vi "breakout.vi"(11 "NXT/EV3":T1) -> (3 "NXT/EV3 2":T1)   [LabVIEW 2013]
uses:
  <vilib>/NXT/Subs/LVHSConnector.ctl
  <vilib>/NXT/LegoClasses/BrickReference/BrickReference.lvclass
  <vilib>/NXT/Dual Mode Library/Display/NXT_Rect.ctl
  <vilib>/NXT/Dual Mode Library/Display/clearDisplay.vi
  <vilib>/NXT/Dual Mode Library/Waits/Wait_Num.vi
  <vilib>/NXT/Dual Mode Library/prims/inRangeAndCoerce/inRangeAndCoerce_float.vi
  <vilib>/NXT/Dual Mode Library/Display/eraseRect.vi
  <vilib>/NXT/Dual Mode Library/Display/drawRect_filled.vi
  <vilib>/NXT/Dual Mode Library/Advanced/NXTFlag_Get_Integer.vi
  <vilib>/NXT/Dual Mode Library/Sensors/EV3_Infrared_Seek.vi
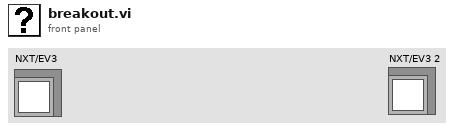
[diagram p1: front panel]
types:
  T1 = typedef "LVHSConnector.ctl" = refnum<class "BrickReference.lvclass">
  T2 = typedef "NXT_Rect.ctl" = cluster{"Left":i16, "Bottom":i16, "Width":i16, "Height":i16}
  T3 = cluster{dbl, dbl, "lower limit":i32, "lower limit":i32}
  T4 = cluster{"Channel 1 Heading":sgl, "Channel 1 Proximity":sgl, "Channel 2 Heading":sgl, "Channel 2 Proximity":sgl, "Channel 3 Heading":sgl, "Channel 3 Proximity":sgl, "Channel 4 Heading":sgl, "Channel 4 Proximity":sgl}
  T5 = cluster{sgl, "Start  Y":i16, "Start  Y":i16, "Start  Y":i16}
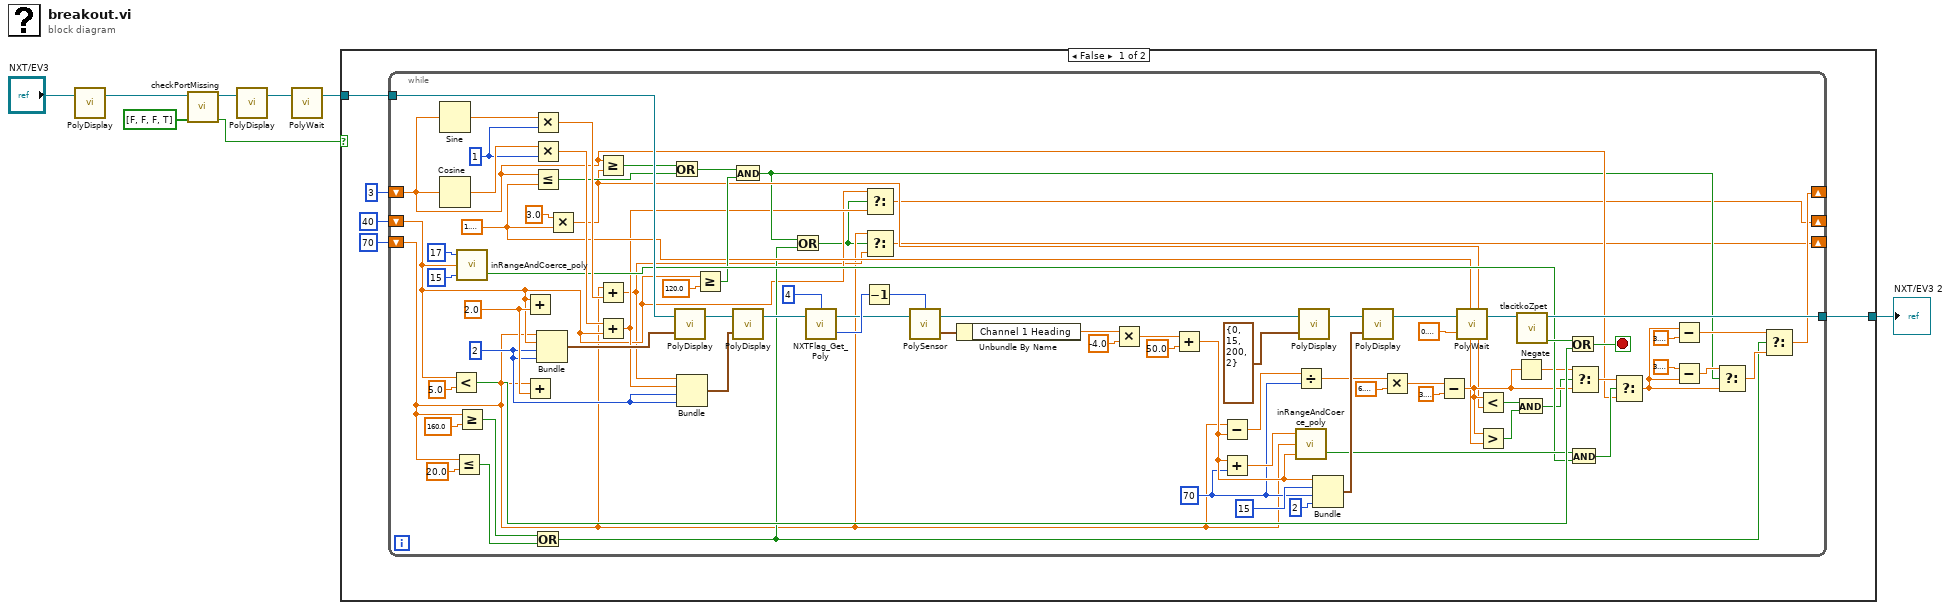
[diagram p0: block diagram]
diagram:
  n1 = call-poly <vilib>:"PolyDisplay.vi"("NXT/EV3"="NXT/EV3") -> ("NXT/EV3"=w7:T1)  [unwired: 3 in]
  n2 = call "checkPortMissing.vi"("Required"=bool[] [FALSE, FALSE, FALSE, TRUE], "NXT/EV3"=w7) -> ("Success"=w5:bool, "NXT/EV3"=w3:T1)  [unwired: 8 in]
  n3 = call-poly <vilib>:"PolyDisplay.vi"("NXT/EV3"=w3) -> ("NXT/EV3"=w1:T1)  [unwired: 3 in]
  n4 = call-poly <vilib>:"PolyWait.vi"("NXT/EV3"=w1) -> ("NXT/EV3"=w2:T1)  [unwired: 3 in]
  n5 = case shown="False" w5 {
    tunnel: [w12 w97] -> w4
    tunnel: w2 -> [w13 w97]
    frame False {
      n6 = while {
        tunnel: w13 -> [w67]
        tunnel: [w59] -> w12
        shift-right: [w26] -> _
        shift-left: 3 -> [w32]
        shift-right: [w16] -> _
        shift-left: 70 -> [w15]
        shift-right: [w19] -> _
        shift-left: 40 -> [w18]
        stop <- w61 stop-if-true
        w28 = 2 ("lower limit")
        w30 = 1.5707963267948966
        w54 = i16 70 ("Start  Y")
        w72 = 2.0
        w74 = 1
        n7 = Sine(x=w32) -> (sin(x)=w78:dbl)
        n8 = Cosine(x=w32) -> (cos(x)=w77:dbl)
        n9 = Less?(x=w18, y=5.0) -> (x < y?=w62:bool)
        n10 = Less Or Equal?(x=w15, y=20.0) -> (x <= y?=w39:bool)
        n11 = call-poly <vilib>:"inRangeAndCoerce_poly.vi"("lower limit"=15, "x"=w18, "upper limit"=17) -> ("In Range?"=w51:bool)  [unwired: 1 out]
        n12 = Greater Or Equal?(x=w15, y=160.0) -> (x >= y?=w41:bool)
        n13 = Add(x=w18, y=w72) -> ()  [unwired: 1 out]
        n14 = Add(x=w15, y=w72) -> ()  [unwired: 1 out]
        n15 = Multiply(x=w78, y=w74) -> (x*y=w76:dbl)
        n16 = Multiply(x=w77, y=w74) -> (x*y=w75:dbl)
        n17 = Less Or Equal?(x=w32, y=w30) -> (x <= y?=w33:bool)
        n18 = Or(x=w41, y=w39) -> (x .or. y?=w21:bool)
        n19 = Bundle(w15, w18, "lower limit"=w28, "lower limit"=w28) -> (w68:T3)  [unwired: 1 in]
        n20 = Multiply(x=3.0, y=w30) -> (x*y=w31:dbl)
        n21 = Greater Or Equal?(x=w32, y=w31) -> (x >= y?=w35:bool)
        n22 = Add(x=w15, y=w76) -> (x+y=w17:dbl)
        n23 = Add(x=w75, y=w18) -> (x+y=w20:dbl)
        n24 = Or(x=w35, y=w33) -> (x .or. y?=w34:bool)
        n25 = call-poly <vilib>:"PolyDisplay.vi"("Rect Parameters"=w68, "NXT/EV3"=w67) -> ("NXT/EV3"=w66:T1)  [unwired: 2 in]
        n26 = Bundle(w17, w20, "lower limit"=w28, "lower limit"=w28) -> (w84:T3)  [unwired: 1 in]
        n27 = Greater Or Equal?(x=w18, y=120.0) -> (x >= y?=w38:bool)
        n28 = And(x=w34, y=w38) -> (x .and. y?=w22:bool)
        n29 = call-poly <vilib>:"PolyDisplay.vi"("Rect Parameters"=w84, "NXT/EV3"=w66) -> ("NXT/EV3"=w83:T1)  [unwired: 2 in]
        n30 = Or(x=w22, y=w21) -> (x .or. y?=w14:bool)
        n31 = call-poly <vilib>:"NXTFlag_Get_Poly.vi"("NXT/EV3"=w83, "NXT/EV3 Flag Number"=4) -> ("Flag Value"=w95:i32, "NXT/EV3"=w94:T1)  [unwired: 1 in]
        n32 = Decrement(x=w95) -> (x-1=w93:i32)
        n33 = Select(t=w18, s=w14, f=w20) -> (s? t:f=w19:dbl)
        n34 = Select(t=w15, s=w14, f=w17) -> (s? t:f=w16:dbl)
        n35 = call-poly <vilib>:"PolySensor.vi"("NXT/EV3"=w94, "Port (Port 1)"=w93) -> ("Scaled Values"=w92:T4, "NXT/EV3"=w89:T1)  [unwired: 1 in]
        n36 = Unbundle By Name(w92) -> ("Channel 1 Heading"=w91:sgl)
        n37 = Multiply(x=w91, y=sgl -4.0) -> (x*y=w86:sgl)
        n38 = Add(x=w86, y=sgl 50.0) -> (x+y=w55:sgl)
        n39 = Subtract(x=w15, y=w55) -> (x-y=w82:dbl)
        n40 = Add(x=w55, y=w54) -> (x+y=w56:sgl)
        n41 = Divide(x=w82, y=w54) -> (x/y=w80:dbl)
        n42 = call-poly <vilib>:"inRangeAndCoerce_poly.vi"("lower limit"=w55, "x"=w15, "upper limit"=w56) -> ("In Range?"=w53:bool)  [unwired: 1 out]
        n43 = call-poly <vilib>:"PolyDisplay.vi"("Rect Parameters"=T2 {"Left"=0, "Bottom"=15, "Width"=200, "Height"=2}, "NXT/EV3"=w89) -> ("NXT/EV3"=w88:T1)  [unwired: 2 in]
        n44 = Bundle(w55, "Start  Y"=i16 15, "Start  Y"=w54, "Start  Y"=i16 2) -> (w90:T5)  [unwired: 1 in]
        n45 = call-poly <vilib>:"PolyDisplay.vi"("Rect Parameters"=w90, "NXT/EV3"=w88) -> ("NXT/EV3"=w52:T1)  [unwired: 2 in]
        n46 = Multiply(x=w80, y=6.283185307179586) -> (x*y=w79:dbl)
        n47 = Subtract(x=w79, y=3.141592653589793) -> (x-y=w47:dbl)
        n48 = call-poly <vilib>:"PolyWait.vi"("Time (1 sec)"=sgl 0.1, "NXT/EV3"=w52) -> ("NXT/EV3"=w60:T1)  [unwired: 2 in]
        n49 = Less?(x=w47, y=w31) -> (x < y?=w45:bool)
        n50 = Greater?(x=w47, y=w30) -> (0:w46:bool)
        n51 = Negate(x=w47) -> (-x=w49:dbl)
        n52 = And(x=w45, y=w46) -> (x .and. y?=w44:bool)
        n53 = call "tlacitkoZpet.vi"("NXT/EV3"=w60) -> ("Boolean"=w58:bool, "NXT/EV3 2"=w59:T1)  [unwired: 9 in]
        n54 = Or(x=w58, y=w62) -> (x .or. y?=w61:bool)
        n55 = And(x=w53, y=w51) -> (x .and. y?=w50:bool)
        n56 = Select(t=w49, s=w44, f=w47) -> (s? t:f=w48:dbl)
        n57 = Select(t=w48, s=w50, f=w32) -> (s? t:f=w24:dbl)
        n58 = Subtract(x=w24, y=3.141592653589793) -> (x-y=w25:dbl)
        n59 = Subtract(x=3.141592653589793, y=w24) -> (x-y=w29:dbl)
        n60 = Select(t=w29, s=w22, f=w24) -> (s? t:f=w27:dbl)
        n61 = Select(t=w25, s=w21, f=w27) -> (s? t:f=w26:dbl)
      }
    }
    frame True {
      # "Controllers unavailable"
    }
  }
  "NXT/EV3 2" <- w4
